vi "Convert String to Timestamp.vi"() -> ()   [LabVIEW 2013]
panel:
  out "Time Stamp":timestamp
  in  "Timestamp String":string
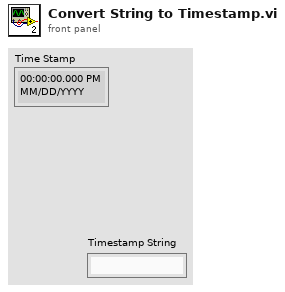
[diagram p1: front panel]
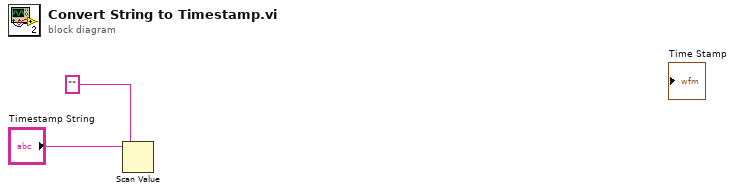
[diagram p0: block diagram]
diagram:
  n1 = Scan Value(string="Timestamp String", format string="") -> ()  [unwired: 1 in, 2 out]
